vi "Unpack Menu Selection.vi"(11 "MenuSelectionMsg":refnum<class "MenuSelectionMsg.lvclass">) -> (0 "Item Tag":string, 1 "Time":u32, 2 "MenuRef":refnum<k9>, 3 "VI Refnum":refnum<vi>, 4 "Item Path":string, 5 "App Item?":bool)   [LabVIEW 2015, in "ActorEvents.lvlib" / "MenuSelectionMsg.lvclass"]
doc: "<License>\nCopyright © 2017 Composed Systems, LLC | All rights reserved\nwww.composed.io\n\nAuthor: Ethan Stern <ethan.stern@composed.io>\n\nThis software is provided \"AS IS\" WITHOUT WARRANTIES, either express or implied, AND IS FOR EDUCATIONAL PURPOSES ONLY.\n</License>"
uses:
  MenuSelectionMsg.lvclass
  MenuSelectionMsg.lvclass/MenuSelectionMsg.ctl
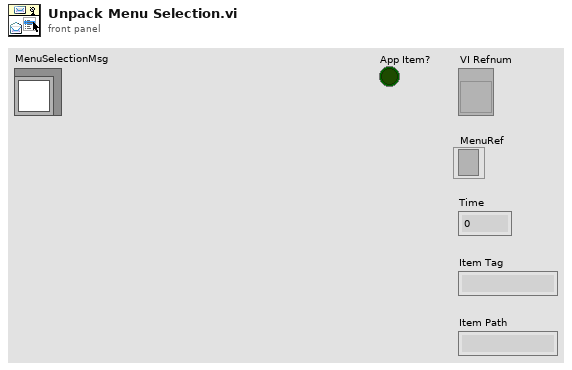
[diagram p1: front panel]
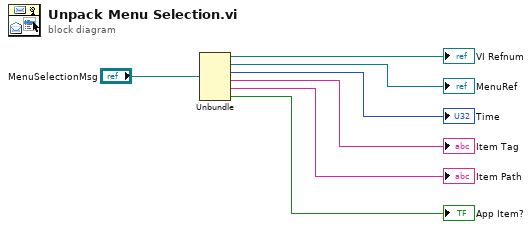
[diagram p0: block diagram]
diagram:
  n1 = Unbundle("MenuSelectionMsg") -> (→"VI Refnum":refnum<vi>, →"MenuRef":refnum<k9>, →"Time":u32, →"Item Tag":string, →"Item Path":string, →"App Item?":bool)
